vi "Peregrine_read_parameters.vi"(0 "Handle in":refnum<visa-resource-name>, 2 "Address":u8, 7 "Select parameter":T1(ring), 11 "error":errorcluster) -> (4 "Handle out":refnum<visa-resource-name>, 6 "Key response":u32, 10 "Value response":i32, 15 "error out":errorcluster)   [LabVIEW 2019]
panel:
  # "Inputs"
  # "Response message"
  # "Output"
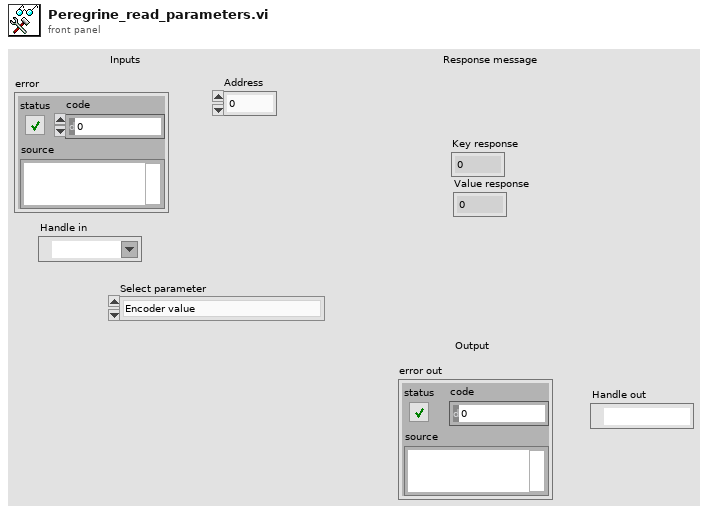
[diagram p1: front panel]
types:
  T1 = enum16{"Encoder value", "Operating mode", "Path planning mode", "Encoder mode", "Microstepping mode", "Limit switch mode", "Control mode", "Power save mode", "Read firmware version", "Read driver uptime"}
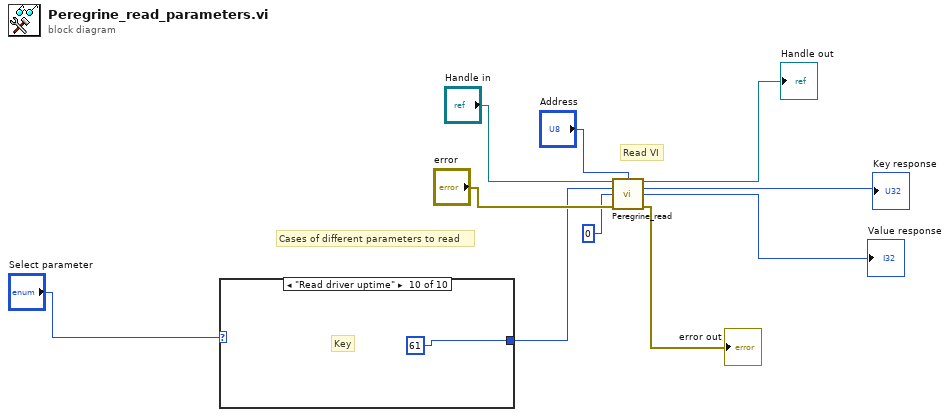
[diagram p0: block diagram]
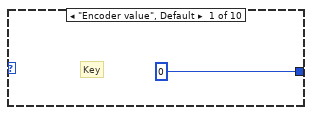
[diagram p2: hidden frame]
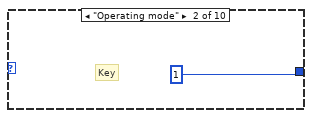
[diagram p3: hidden frame]
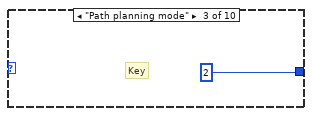
[diagram p4: hidden frame]
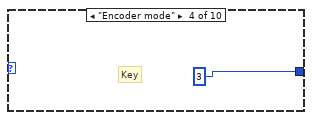
[diagram p5: hidden frame]
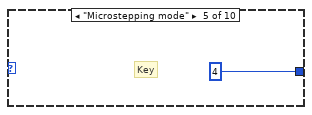
[diagram p6: hidden frame]
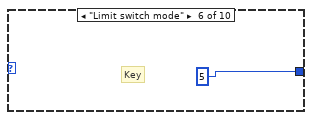
[diagram p7: hidden frame]
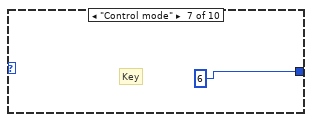
[diagram p8: hidden frame]
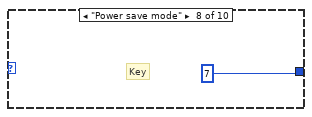
[diagram p9: hidden frame]
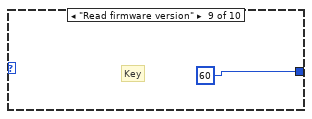
[diagram p10: hidden frame]
diagram:
  # "Cases of different parameters to read"
  # "Read VI"
  n1 = case shown="\"Read driver uptime\"" "Select parameter" {
    tunnel: [u32 0 u32 1 u32 2 u32 3 u32 4 u32 5 u32 6 u32 7 u32 60 u32 61] -> w1
    frame "Encoder value", Default {
      # "Key"
    }
    frame "Operating mode" {
      # "Key"
    }
    frame "Path planning mode" {
      # "Key"
    }
    frame "Encoder mode" {
      # "Key"
    }
    frame "Microstepping mode" {
      # "Key"
    }
    frame "Limit switch mode" {
      # "Key"
    }
    frame "Control mode" {
      # "Key"
    }
    frame "Power save mode" {
      # "Key"
    }
    frame "Read firmware version" {
      # "Key"
    }
    frame "Read driver uptime" {
      # "Key"
    }
  }
  n2 = call "Peregrine_read.vi"("Handle in"="Handle in", "Address"="Address", "Key"=w1, "Value"=0, "error"="error") -> ("Handle out"=→"Handle out":refnum<visa-resource-name>, "Key response"=→"Key response":u32, "Value response"=→"Value response":i32, "error out"=→"error out":errorcluster)  [unwired: 7 in]
